vi "Get AI names from PGserver.vi"(6 "conn":T2={"host"="localhost", "port"="5432", "client_encoding"="WIN1251", "dbname"="data", "user"="postgres", "password"=""}, 8 "error in (no error)":errorcluster, 9 "AIParamColumns":string[](array[string])=["fcode_full", "fname", "process_units"], 10 "AIParamTable":string="fa_3", 11 "AIParameters":string[](array[string])) -> (0 "error out":errorcluster, 3 "Names table":string[][](array[string]))   [LabVIEW 2019, in "Inputs.lvlib"]
uses:
  Inputs.lvlib
  Database/ctl/Coninfo.ctl
  Database/PostgreSQL2LabVIEW/libpqlv/src/PQfinish.vi
  Database/PostgreSQL2LabVIEW/libpqlv/src/PQconnectdb.vi
  Database/PostgreSQL2LabVIEW/libpqlv/src/PQerrorMessage.vi
  Database/PostgreSQL2LabVIEW/libpqlv/src/PQstatus.vi
  <vilib>/dlg_ctls.llb/Space Constant.vi
  Database/Progress.vi
  Database/PostgreSQL.lvlib
  Database/PostgreSQL2LabVIEW/libpqUtility64/libpqutility64.lvlib
  Database/PostgreSQL2LabVIEW/libpqUtility/libpqutility.lvlib
panel:
  out "PQStatus":T1(ring)
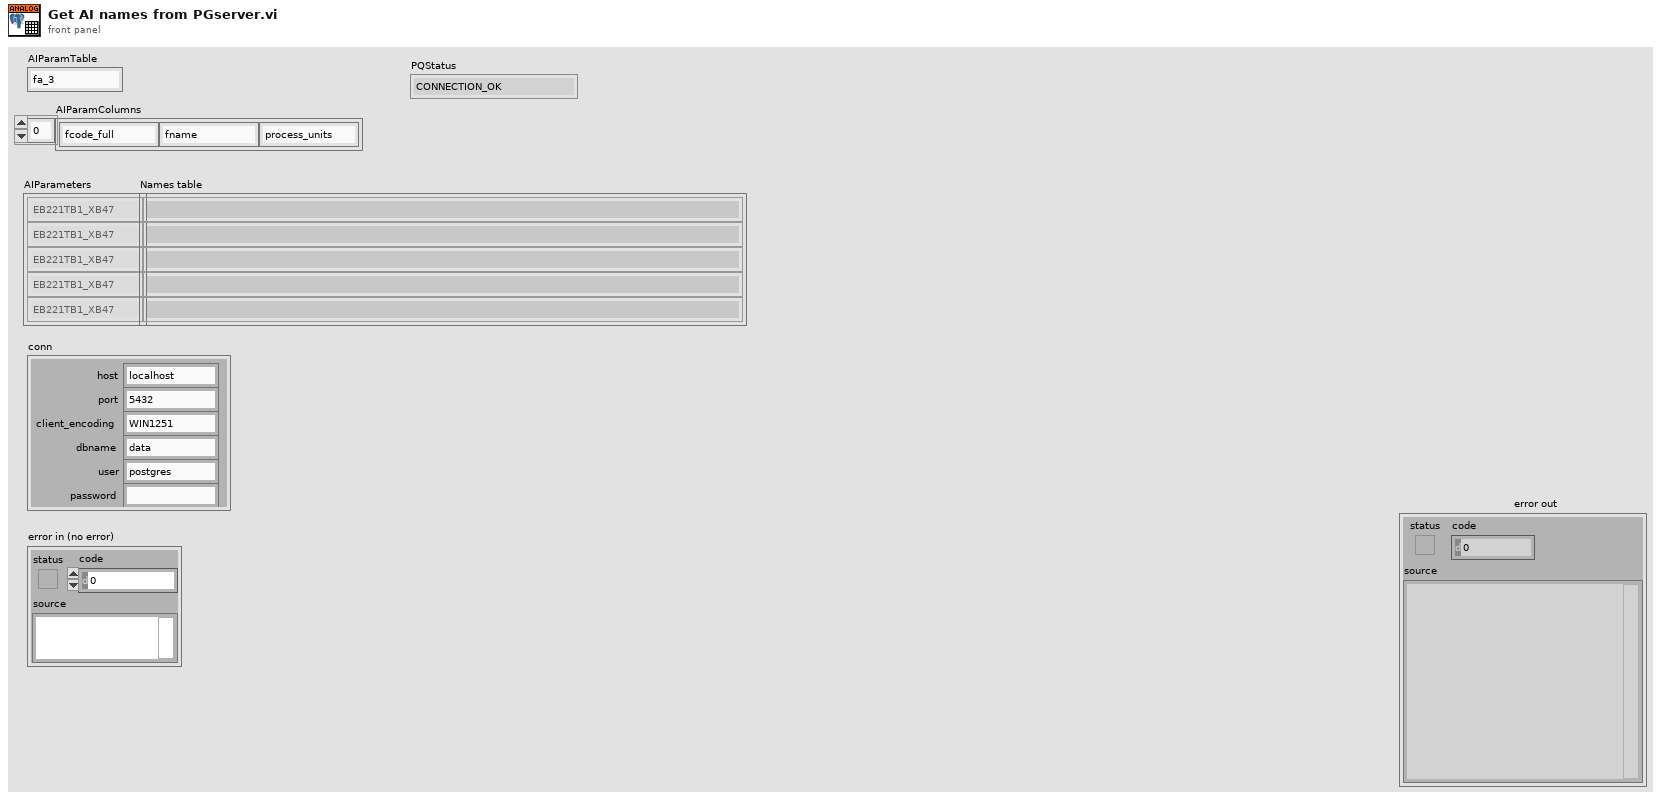
[diagram p1: front panel]
types:
  T1 = enum32{"CONNECTION_OK", "CONNECTION_BAD", "CONNECTION_STARTED", "CONNECTION_MADE", "CONNECTION_AWAITING_RESPONSE", "CONNECTION_AUTH_OK", "CONNECTION_SETENV", "CONNECTION_SSL_STARTUP", "CONNECTION_NEEDED"}
  T2 = typedef "PostgreSQL.lvlib/Coninfo.ctl" = cluster{"host":string, "port":string, "client_encoding":string, "dbname":string, "user":string, "password":string}
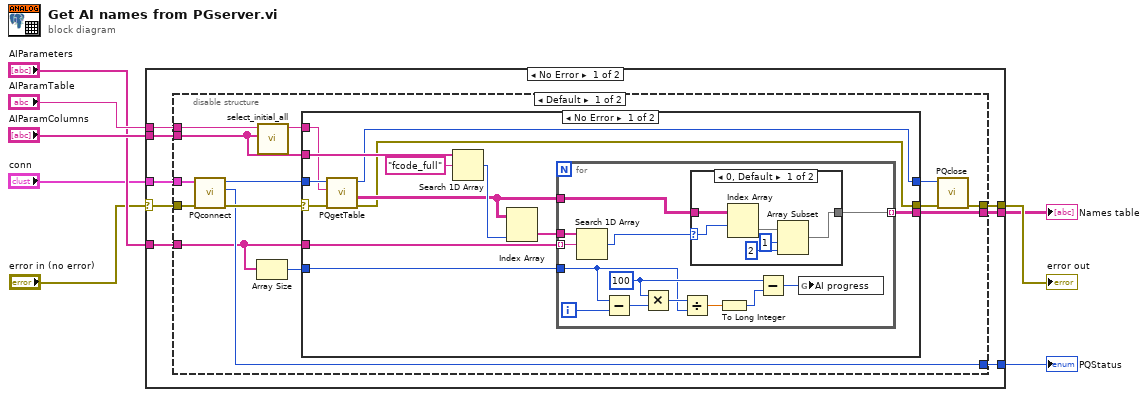
[diagram p0: block diagram]
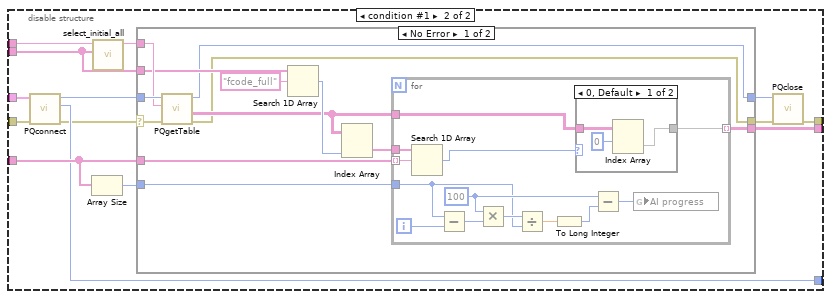
[diagram p4: hidden frame]
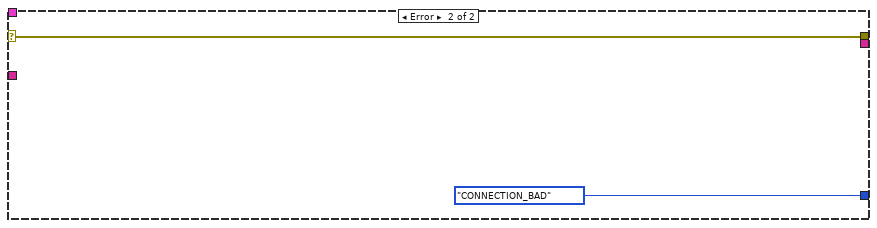
[diagram p7: hidden frame]
diagram:
  n1 = case shown="No Error" "error in (no error)" {
    selector: "error in (no error)" -> [w11 w111]
    tunnel: [w16 w111] -> w8
    tunnel: [w15 _] -> w7
    tunnel: "AIParamColumns" -> [w14 _]
    tunnel: "conn" -> [w10 _]
    tunnel: "AIParamTable" -> [w13 _]
    tunnel: "AIParameters" -> [w12 _]
    tunnel: [w9 T1."CONNECTION_BAD" ("PQStatus")] -> w1
    frame No Error {
      n2 = disable-structure shown="Default" {
        disable-tunnel: [w17 w65] -> w16
        disable-tunnel: [w24 w73] -> w15
        disable-tunnel: w14 -> [w20 w75]
        disable-tunnel: w13 -> [w22 w76]
        disable-tunnel: w12 -> [w23 w74]
        disable-tunnel: w11 -> [w26 w71]
        disable-tunnel: w10 -> [w27 w72]
        disable-tunnel: [w25 w69] -> w9
        frame condition #0 (active) {
          n3 = call "PQconnect.vi"("error in (no error)"=w26, "conninfo"=w27) -> ("error out"=w28:errorcluster, "PQStatus"=w25:T1, "conn"=w29:u32)  [unwired: 7 in]
          n4 = Array Size(array=w23) -> (size(s)=w30:i32)
          n5 = call "select_initial_all.vi"("Column table"=w20, "table"=w22) -> ("parameters"=w21:string)  [unwired: 8 in, 1 out]
          n6 = case shown="No Error" w28 {
            selector: w28 -> [w35 w63]
            tunnel: w30 -> [w43 _]
            tunnel: w21 -> [w34 _]
            tunnel: [w31 w63] -> w18
            tunnel: [w33 w64] -> w19
            tunnel: [w42 _] -> w24
            tunnel: w29 -> [w36 w64]
            tunnel: w23 -> [w38 _]
            tunnel: w20 -> [w37 _]
            frame No Error {
              n7 = call "PQgetTable.vi"("error in"=w35, "query"=w34, "conn"=w36) -> ("error out"=w31:errorcluster, "Data"=w32:string[][], "conn_out"=w33:u32)  [unwired: 4 in, 2 out]
              n8 = Search 1D Array(1D array=w37, element="fcode_full" ("table")) -> (index of element=w40:i32)  [unwired: 1 in]
              n9 = Index Array(array=w32, index (col)=w40) -> (element=w39:string[])  [unwired: 1 in]
              n10 = for {
                tunnel: w43 -> [w49]
                tunnel: [w48] -> w42 mode=indexing
                tunnel: w39 -> [w47]
                tunnel: w38 -> [w46] mode=indexing
                tunnel: w32 -> [w44]
                i -> [w50]
                w54 = 100 ("y")
                n11 = Search 1D Array(1D array=w47, element=w46) -> (index of element=w45:i32)  [unwired: 1 in]
                n12 = Subtract(x=w49, y=w50) -> (x-y=w53:i32)
                n13 = Multiply(x=w54, y=w53) -> (x*y=w56:i32)
                n14 = Divide(x=w56, y=w49) -> (x/y=w52:dbl)
                n15 = case shown="0, Default" w45 {
                  selector: w45 -> [w61 _]
                  tunnel: w44 -> [w62 _]
                  tunnel: [w59 _] -> w48
                  frame 0, Default {
                    n16 = Index Array(array=w62, index (row)=w61) -> (element=w60:string[])  [unwired: 1 in]
                    n17 = Array Subset(array=w60, index=1, length=2) -> (w59:string[])
                  }
                  frame -1 {
                  }
                }
                n18 = To Long Integer(number=w52) -> (32bit integer=w51:i32)
                n19 = Subtract(x=w54, y=w51) -> (x-y=w55:i32)
                n20 = global write "Progress.vi" "AI progress"(w55) -> ()
              }
            }
            frame Error {
            }
          }
          n21 = call "PQclose.vi"("error in (no error)"=w18, "conn"=w19) -> ("error out"=w17:errorcluster)  [unwired: 9 in]
        }
        frame condition #1 {
          n22 = call "PQconnect.vi"("error in (no error)"=w71, "conninfo"=w72) -> ("error out"=w68:errorcluster, "PQStatus"=w69:T1, "conn"=w70:u64)  [unwired: 7 in]
          n23 = Array Size(array=w74) -> (size(s)=w78:i32)
          n24 = call "select_initial_all.vi"("Column table"=w75, "table"=w76) -> ("parameters"=w77:string)  [unwired: 8 in, 1 out]
          n25 = case shown="No Error" w68 {
            selector: w68 -> [w79 w108]
            tunnel: w78 -> [w91 _]
            tunnel: w77 -> [w83 _]
            tunnel: [w81 w108] -> w66
            tunnel: [w80 w109] -> w67
            tunnel: [w90 _] -> w73
            tunnel: w70 -> [w84 w109]
            tunnel: w74 -> [w86 _]
            tunnel: w75 -> [w82 _]
            frame No Error {
              n26 = call "PQgetTable.vi"("error in"=w79, "query"=w83, "conn"=w84) -> ("error out"=w81:errorcluster, "Data"=w85:string[][], "conn_out"=w80:u64)  [unwired: 4 in, 2 out]
              n27 = Search 1D Array(1D array=w82, element="fcode_full" ("table")) -> (index of element=w88:i32)  [unwired: 1 in]
              n28 = Index Array(array=w85, index (col)=w88) -> (element=w87:string[])  [unwired: 1 in]
              n29 = for {
                tunnel: w91 -> [w97]
                tunnel: [w96] -> w90 mode=indexing
                tunnel: w87 -> [w95]
                tunnel: w86 -> [w94] mode=indexing
                tunnel: w85 -> [w92]
                i -> [w98]
                w102 = 100 ("y")
                n30 = Search 1D Array(1D array=w95, element=w94) -> (index of element=w93:i32)  [unwired: 1 in]
                n31 = Subtract(x=w97, y=w98) -> (x-y=w101:i32)
                n32 = Multiply(x=w102, y=w101) -> (x*y=w104:i32)
                n33 = Divide(x=w104, y=w97) -> (x/y=w100:dbl)
                n34 = To Long Integer(number=w100) -> (32bit integer=w99:i32)
                n35 = case shown="0, Default" w93 {
                  tunnel: w92 -> [w106 _]
                  tunnel: [w105 _] -> w96
                  frame 0, Default {
                    n36 = Index Array(array=w106, index (row)=0) -> (element=w105:string[])  [unwired: 1 in]
                  }
                  frame -1 {
                  }
                }
                n37 = Subtract(x=w102, y=w99) -> (x-y=w103:i32)
                n38 = global write "Progress.vi" "AI progress"(w103) -> ()
              }
            }
            frame Error {
            }
          }
          n39 = call "PQclose.vi"("error in (no error)"=w66, "conn"=w67) -> ("error out"=w65:errorcluster)  [unwired: 9 in]
        }
      }
    }
    frame Error {
    }
  }
  "error out" <- w8
  "Names table" <- w7
  "PQStatus" <- w1
